vi "Connect.vi"(8 "error in (no error)":errorcluster, 11 "FTPProtocol in":refnum<class "FTPProtocol.lvclass">) -> (0 "error out":errorcluster, 1 "Connected?":bool=TRUE, 3 "FTPProtocol out":refnum<class "FTPProtocol.lvclass">)   [LabVIEW 2020, in "CSM-FileSync.lvlib" / "FTPProtocol.lvclass"]
uses:
  FTPProtocol.lvclass
  FTPProtocol.lvclass/FTPProtocol.ctl
  FTP Toolkit/FTP Class/FTP.lvclass
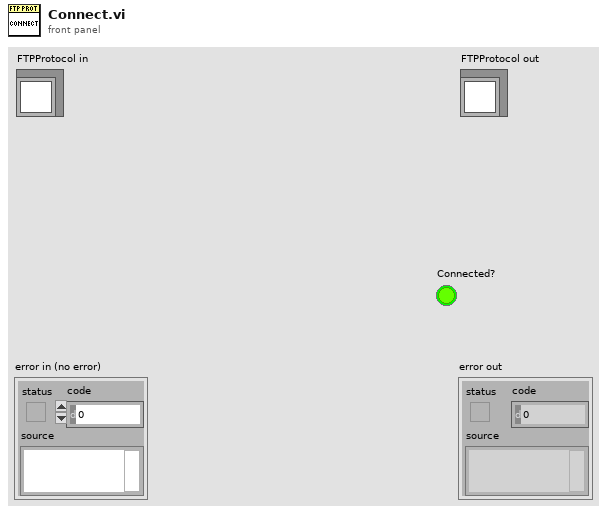
[diagram p1: front panel]
types:
  T1 = cluster{"address":string, "remote port":u16, "userName":string, "passWord":string, "RootDir":string}
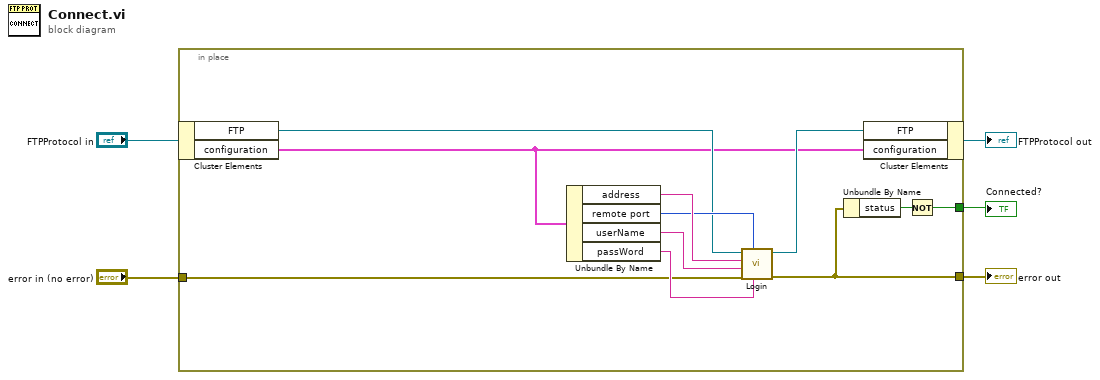
[diagram p0: block diagram]
diagram:
  n1 = in-place {
    in-place-border: "error in (no error)" -> [w7]
    in-place-border: [w9] -> w4
    in-place-border: [w8] -> w1
    n2 = in-place-cluster #1("FTPProtocol in") -> ("FTP"=w11:refnum<class "FTP.lvclass">, "configuration"=w6:T1)
    n3 = Unbundle By Name(w6) -> ("address"=w16:string, "remote port"=w15:u16, "userName"=w14:string, "passWord"=w13:string)
    n4 = call "Login.vi"("passWord"=w13, "remote port (21)"=w15, "error in (no error)"=w7, "userName"=w14, "address"=w16, "FTP in"=w11) -> ("error out"=w9:errorcluster, "FTP out"=w12:refnum<class "FTP.lvclass">)  [unwired: 4 in]
    n5 = Unbundle By Name(w9) -> ("status"=w10:bool)
    n6 = in-place-cluster #1("FTP"=w12, "configuration"=w6) -> (→"FTPProtocol out":refnum<class "FTPProtocol.lvclass">)
    n7 = Not(x=w10) -> (.not. x?=w8:bool)
  }
  "error out" <- w4
  "Connected?" <- w1
